vi "SSC DCPower Configure Aperture Time.vi"(0 "DCPower SSC in":T1[](array[typedef]), 5 "Aperture Time":dbl format="%#_6p", 7 "Aperture Time Units":T2=1028 caption="aperture time units" items=["Seconds"=1028, "Powerline Cycles"=1029], 11 "error in":errorcluster) -> (4 "DCPower SSC out":T1[](array[typedef]), 15 "error out":errorcluster)   [LabVIEW 2020]
doc: "This VI configures measurement aperture time of the sessions."
uses:
  <instrlib>/niDCPower/nidcpower.llb/niDCPower Aperture Time Units.ctl
  SSC DCPower.ctl
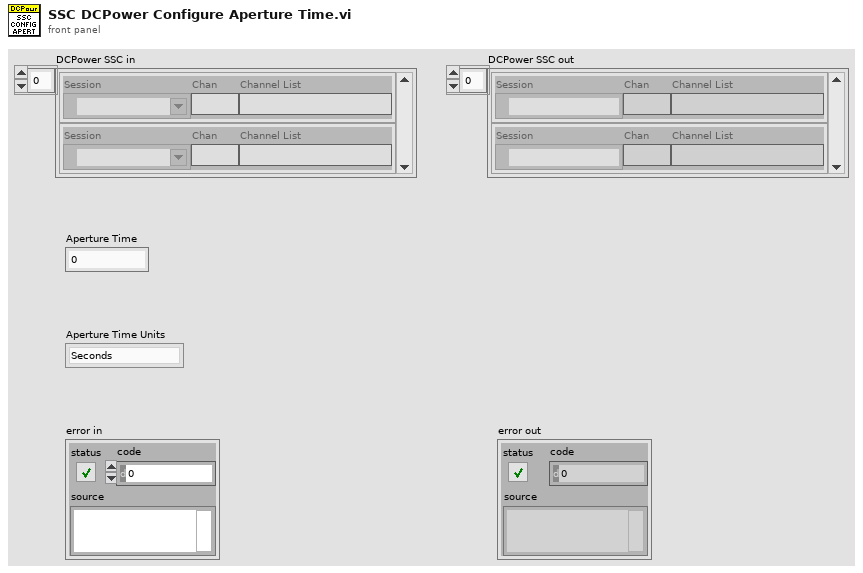
[diagram p1: front panel]
types:
  T1 = typedef "SSC DCPower.ctl" = cluster{"Session":refnum<k15>, "Chan":string, "Channel List":string}
  T2 = typedef "niDCPower Aperture Time Units.ctl" = i32
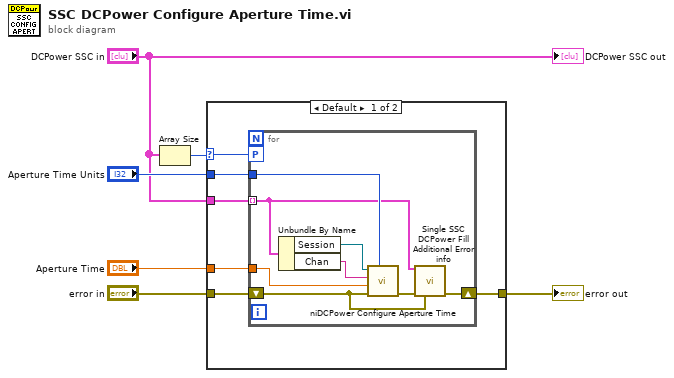
[diagram p0: block diagram]
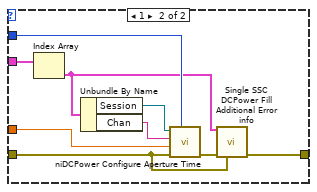
[diagram p2: hidden frame]
diagram:
  n1 = Array Size(array="DCPower SSC in") -> (size(s)=w2:i32)
  n2 = case shown="Default" w2 {
    selector: w2 -> [w8 _]
    tunnel: "error in" -> [w12 w29]
    tunnel: "Aperture Time Units" -> [w11 w28]
    tunnel: "Aperture Time" -> [w10 w27]
    tunnel: [w9 w26] -> w3
    tunnel: "DCPower SSC in" -> [w7 w25]
    frame Default {
      n3 = for {
        tunnel: w7 -> [w14] mode=indexing
        workers-P: w8 -> [_]
        tunnel: w11 -> [w19]
        tunnel: w10 -> [w20]
        shift-right: [w15] -> w9
        shift-left: w12 -> [w13]
        n4 = Unbundle By Name(w14) -> ("Session"=w17:refnum<k15>, "Chan"=w16:string)
        n5 = call <instrlib>:"niDCPower Configure Aperture Time.vi"("aperture time units"=w19, "error in (no error)"=w13, "aperture time"=w20, "channel name"=w16, "instrument handle"=w17) -> ("error out"=w18:errorcluster)  [unwired: 5 in, 1 out]
        n6 = call "Single SSC DCPower Fill Additional Error info.vi"("DCPower SSC in"=w14, "error in"=w18, "previous error in"=w13) -> ("error out"=w15:errorcluster)  [unwired: 12 in]
      }
    }
    frame 1 {
      n7 = Index Array(array=w25) -> (element=w21:T1)  [unwired: 1 in]
      n8 = Unbundle By Name(w21) -> ("Session"=w23:refnum<k15>, "Chan"=w22:string)
      n9 = call <instrlib>:"niDCPower Configure Aperture Time.vi"("aperture time units"=w28, "error in (no error)"=w29, "aperture time"=w27, "channel name"=w22, "instrument handle"=w23) -> ("error out"=w24:errorcluster)  [unwired: 5 in, 1 out]
      n10 = call "Single SSC DCPower Fill Additional Error info.vi"("DCPower SSC in"=w21, "error in"=w24, "previous error in"=w29) -> ("error out"=w26:errorcluster)  [unwired: 12 in]
    }
  }
  "error out" <- w3
  "DCPower SSC out" <- "DCPower SSC in"
